vi "Chrono.vi"(11 "stop":bool) -> (3 "Sumarized":dbl format="%#_2g")   [LabVIEW 2023]
panel:
  out "Time s":dbl format="%#_2g"
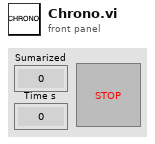
[diagram p1: front panel]
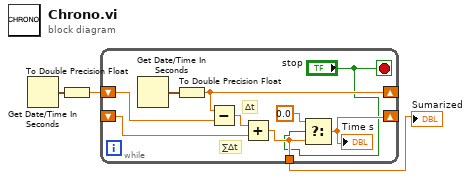
[diagram p0: block diagram]
diagram:
  n1 = Get Date/Time In Seconds() -> (seconds since 1Jan1904=w2:timestamp)
  n2 = To Double Precision Float(number=w2) -> (double precision float=w1:dbl)
  n3 = while {
    shift-right: [w7] -> _
    shift-left: _ -> [w9]
    shift-right: [w6] -> _
    shift-left: w1 -> [w11]
    tunnel: [w5] -> w3
    stop <- "stop" stop-if-true
    # "∑∆t"
    # "∆t"
    n4 = Get Date/Time In Seconds() -> (seconds since 1Jan1904=w12:timestamp)
    n5 = To Double Precision Float(number=w12) -> (double precision float=w6:dbl)
    n6 = Subtract(x=w6, y=w11) -> (x-y=w10:dbl)
    n7 = Add(x=w10, y=w9) -> (x+y=w5:dbl)
    n8 = Select(t=0.0, s="stop", f=w5) -> (s? t:f=w7:dbl)
    "Time s" <- w7
  }
  "Sumarized" <- w3
